vi "FTW-Panel-FrontPanel-SetTitleBar.vi"(0 "Title":string, 1 "VI Refnum":refnum<vi> caption="VI Refnum (Caller)", 11 "error in (no error)":errorcluster) -> (15 "error out":errorcluster)   [LabVIEW 2015]
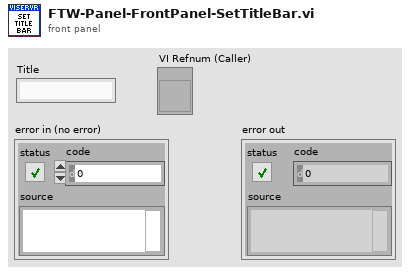
[diagram p1: front panel]
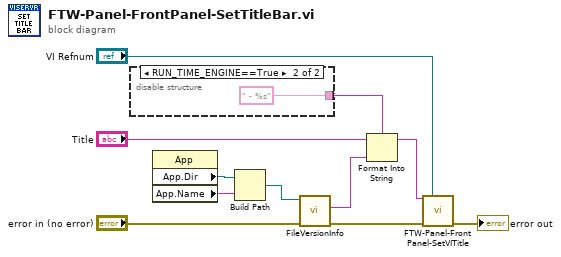
[diagram p0: block diagram]
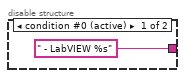
[diagram p2: hidden frame]
diagram:
  n1 = disable-structure shown="RUN_TIME_ENGINE==True" {
    disable-tunnel: [" - LabVIEW %s" ("format string") " - %s" ("format string")] -> w5
    frame condition #0 (active) {
    }
    frame condition #1 {
    }
  }
  n2 = property class="App"() -> ("App.Dir"=w8:path, "App.Name"=w7:string)  [unwired: 2 in, 2 out]
  n3 = Build Path(base path=w8, name or relative path=w7) -> (appended path=w6:path)
  n4 = call <vilib>:"FileVersionInfo.vi"("error in (no error)"="error in (no error)", "Application Path in"=w6) -> ("error out"=w2:errorcluster, "File Version Info"=w4:string)  [unwired: 6 in, 2 out]
  n5 = Format Into String(format string=w5, initial string="Title", w4) -> (resulting string=w1:string)  [unwired: 1 in, 1 out]
  n6 = call "FTW-Panel-FrontPanel-SetVITitle.vi"("Title"=w1, "VI Refnum"="VI Refnum", "error in (no error)"=w2) -> ("error out"=→"error out":errorcluster)  [unwired: 12 in]
